vi "Default_Register_Value_Report.vi"(5 "Default register":u32[](array[numeric])=[6826, 18761, 18761, 18761, 30576, 383, 13312], 7 "input cluster":T1, 8 "error out":errorcluster, 10 "Serial Number":string="testFile", 11 "connection ID":refnum<k5>) -> (0 "error out 2":errorcluster, 3 "connection ID out":refnum<k5>, 4 "Registers Init Value":u32[](array[numeric])=[3413, 6655, 32767, 32767, 16384, 160, 6656])   [LabVIEW 2012]
uses:
  <vilib>/Utility/NIReport.llb/NI_report.lvclass
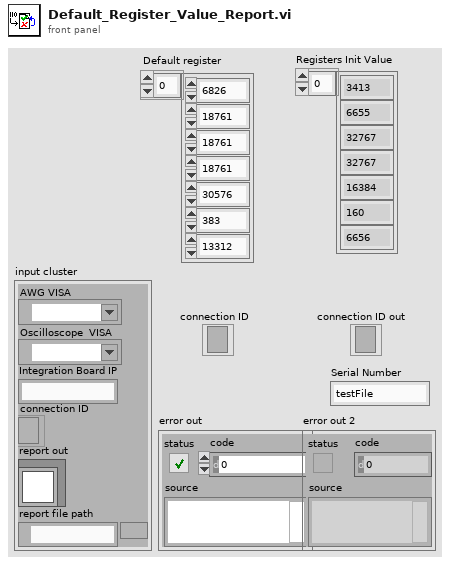
[diagram p1: front panel]
types:
  T1 = cluster{"AWG VISA":refnum<visa-resource-name>, "Oscilloscope  VISA ":refnum<visa-resource-name>, "Integration Board IP":string, "connection ID":refnum<k5>, "report out":refnum<class "NI_report.lvclass">, "report file path":path}
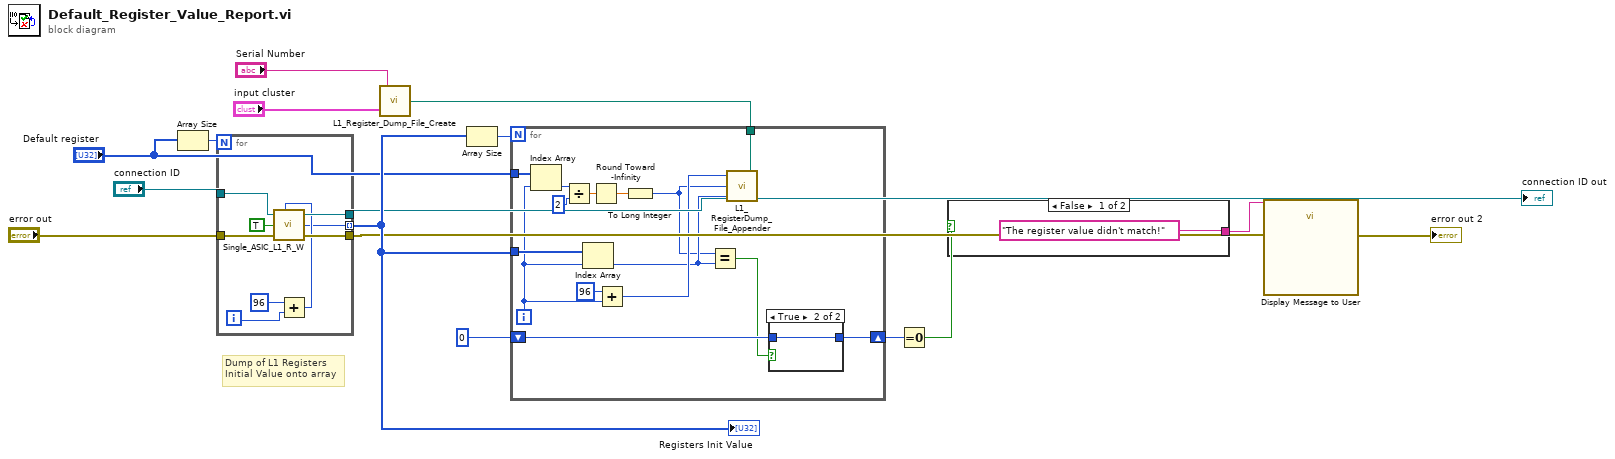
[diagram p0: block diagram]
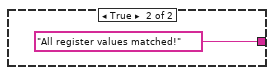
[diagram p2: hidden frame]
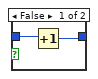
[diagram p3: hidden frame]
diagram:
  # "Dump of L1 Registers\nInitial Value onto array"
  n1 = Array Size(array="Default register") -> (size(s)=w16:i32)
  n2 = for {
    N: w16 -> [_]
    tunnel: "error out" -> [w25]
    tunnel: [w24] -> w12
    tunnel: "connection ID" -> [w23]
    tunnel: [w21] -> w3
    tunnel: [w17] -> w14 mode=indexing
    i -> [w19]
    n3 = Add(x=96 ("y"), y=w19) -> (x+y=w18:i32)
    n4 = call "Single_ASIC_L1_R_W.vi"("connection ID"=w23, "Register or channel"=w18, "RD/#WR"=TRUE, "error in (no error)"=w25) -> ("connection ID out"=w21:refnum<k5>, "data read value"=w17:i64, "error out"=w24:errorcluster)  [unwired: 2 in, 1 out]
  }
  "Registers Init Value" <- w14
  "connection ID out" <- w3
  n5 = call "L1_Register_Dump_File_Create.vi"("input cluster"="input cluster", "Serial Number"="Serial Number") -> ("appended path"=w13:path)
  n6 = Array Size(array=w14) -> (size(s)=w15:i32)
  n7 = for {
    N: w15 -> [_]
    tunnel: w14 -> [w38]
    tunnel: w13 -> [w35]
    tunnel: "Default register" -> [w39]
    shift-right: [w32] -> w10
    shift-left: 0 ("y") -> [w33]
    i -> [w37]
    n8 = Index Array(array=w39, index=w37) -> (element=w29:u32)
    n9 = Divide(x=w29, y=u32 2) -> (x/y=w27:dbl)
    n10 = Index Array(array=w38, index=w37) -> (element=w34:i64)
    n11 = Round Toward -Infinity(1:w27) -> (0:w26:dbl)
    n12 = Add(x=96 ("y"), y=w37) -> (x+y=w36:i32)
    n13 = To Long Integer(number=w26) -> (32bit integer=w30:i32)
    n14 = Equal?(x=w30, y=w34) -> (x = y?=w31:bool)
    n15 = call "L1_RegisterDump_File_Appender.vi"("file path (dialog if empty)"=w35, "Dec Value"=w34, "Register Default"=w30, "Register Number"=w36) -> ()
    n16 = case shown="True" w31 {
      tunnel: w33 -> [w42 w43]
      tunnel: [w41 w43] -> w32
      frame False {
        n17 = Increment(x=w42) -> (x+1=w41:i32)
      }
      frame True {
      }
    }
  }
  n18 = Equal To 0?(x=w10) -> (x = 0?=w9:bool)
  n19 = case shown="False" w9 {
    tunnel: ["The register value didn't match!" ("format string") "All register values matched!" ("format string")] -> w8
    frame False {
    }
    frame True {
    }
  }
  n20 = call "Display Message to User"("error in (no error)"=w12, "Message"=w8) -> ("error out"=→"error out 2":errorcluster)  [unwired: 8 in, 1 out]
